vi "Add Tx Queue Status Section.vi"(8 "error in":errorcluster, 11 "Custom Device Ref in":T1 format="%.0x") -> (0 "error out":errorcluster, 1 "Tx Queue Status channel Refs":T1[](array[typedef]) format="%.0x", 2 "Tx Queue Status Section Ref out":T1 format="%.0x", 3 "Custom Device Ref out":T1 format="%.0x")   [LabVIEW 2020, in "afdx_custom_device Scripting.lvlib"]
uses:
  afdx_custom_device Scripting.lvlib
  <vilib>/NI VeriStand/Custom Device API/Custom Device Item Ref.ctl
  <vilib>/NI VeriStand/Custom Device API/Custom Device Channel.ctl
  <vilib>/NI VeriStand/Custom Device API/Custom Device Channel Type.ctl
  Constants.vi
  <vilib>/NI VeriStand/Custom Device API/Custom Device API.lvlib
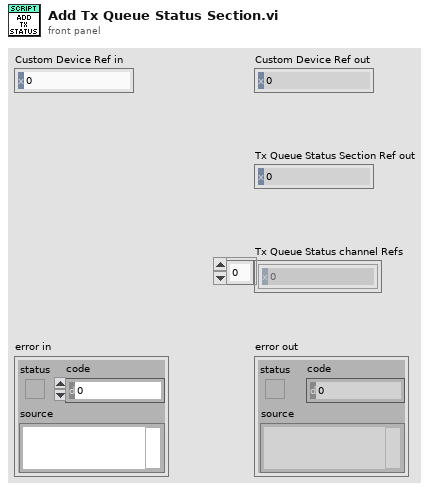
[diagram p1: front panel]
types:
  T1 = typedef "Custom Device API.lvlib/Custom Device Item Ref.ctl" = u64
  T2 = typedef "Custom Device API.lvlib/Custom Device Channel.ctl" = cluster{"Type":T3, "Units":string, "Default Value":dbl, "Faultable":bool, "Scalable":bool}
  T3 = typedef "Custom Device API.lvlib/Custom Device Channel Type.ctl" = enum16{"Input", "Output"}
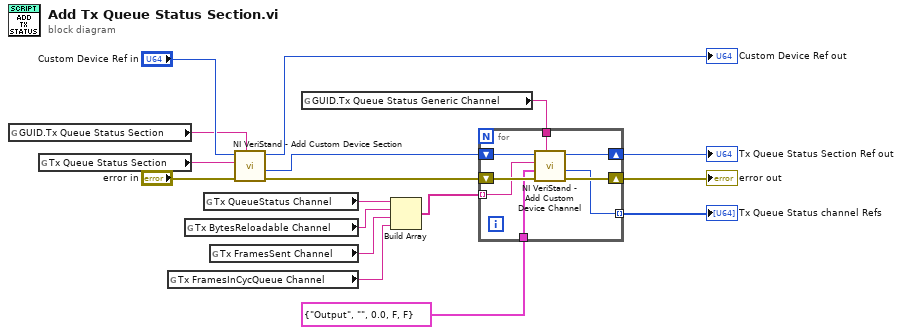
[diagram p0: block diagram]
diagram:
  n1 = global read "Constants.vi" "GUID.Tx Queue Status Section"() -> (w13:string)
  n2 = global read "Constants.vi" "Tx Queue Status Section"() -> (w15:string)
  n3 = global read "Constants.vi" "Tx FramesInCycQueue Channel"() -> (w4:string)
  n4 = global read "Constants.vi" "Tx BytesReloadable Channel"() -> (w6:string)
  n5 = global read "Constants.vi" "Tx QueueStatus Channel"() -> (w7:string)
  n6 = global read "Constants.vi" "Tx FramesSent Channel"() -> (w5:string)
  n7 = call <vilib>:"NI VeriStand - Add Custom Device Section.vi"("GUID (Default Section)"=w13, "error in (no error)"="error in", "Section Name"=w15, "Parent Ref in"="Custom Device Ref in") -> ("error out"=w14:errorcluster, "Section Ptr"=w11:T1, "Parent Ref out"=→"Custom Device Ref out":T1)  [unwired: 4 in, 1 out]
  n8 = global read "Constants.vi" "GUID.Tx Queue Status Generic Channel"() -> (w1:string)
  n9 = Build Array(w7, w6, w5, w4) -> (w3:string[])
  n10 = for {
    tunnel: [w21] -> w8 mode=indexing
    shift-right: [w22] -> w9
    shift-left: w14 -> [w25]
    tunnel: w3 -> [w20] mode=indexing
    tunnel: T2 {"Type"=enum."Output", "Units"="", "Default Value"=0.0, "Faultable"=FALSE, "Scalable"=FALSE} ("Channel") -> [w19]
    tunnel: w1 -> [w18]
    shift-right: [w24] -> w12
    shift-left: w11 -> [w23]
    n11 = call <vilib>:"NI VeriStand - Add Custom Device Channel.vi"("GUID (Default Channel)"=w18, "error in (no error)"=w25, "Channel"=w19, "Channel Name"=w20, "Parent Ref in"=w23) -> ("error out"=w22:errorcluster, "Channel Ref"=w21:T1, "Parent Ref out"=w24:T1)  [unwired: 3 in, 1 out]
  }
  "Tx Queue Status Section Ref out" <- w12
  "error out" <- w9
  "Tx Queue Status channel Refs" <- w8
